vi "Remove Routing and Faulting Custom Device.vi"(8 "error in":errorcluster, 11 "routing and faulting custom device":T1 format="%.0x") -> (0 "error out":errorcluster)   [LabVIEW 2020, in "Routing and Faulting Scripting.lvlib"]
doc: "Removes the Routing and Faulting custom device from its parent. This removes all routing channels and endpoint aliases."
uses:
  Routing and Faulting Scripting.lvlib
  <vilib>/NI VeriStand/Custom Device API/Custom Device Item Ref.ctl
  NationalInstruments.VeriStand.SystemDefinitionAPI
  <vilib>/NI VeriStand/Custom Device API/Custom Device API.lvlib
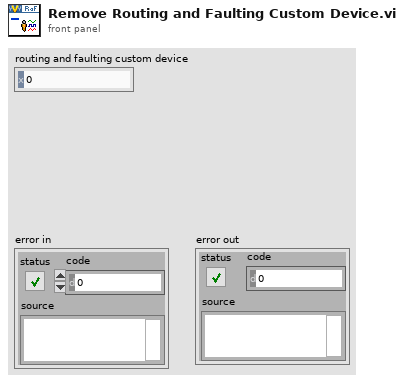
[diagram p1: front panel]
types:
  T1 = typedef "Custom Device API.lvlib/Custom Device Item Ref.ctl" = u64
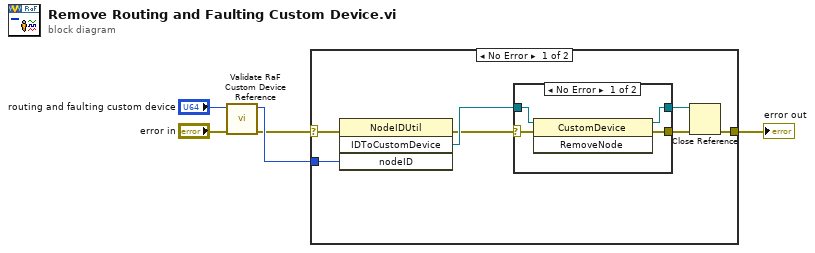
[diagram p0: block diagram]
diagram:
  n1 = call "Validate RaF Custom Device Reference.vi"("error in"="error in", "routing and faulting in"="routing and faulting custom device") -> ("error out"=w1:errorcluster, "routing and faulting out"=w3:T1)  [unwired: 8 in]
  n2 = case shown="No Error" w1 {
    selector: w1 -> [w7 w19]
    tunnel: [w10 w19] -> w5
    tunnel: w3 -> [w8 _]
    frame No Error {
      n3 = invoke class="NodeIDUtil" method="IDToCustomDevice"(error in=w7, "nodeID"=w8) -> (error out=w6:errorcluster, "IDToCustomDevice"=w9:refnum<k24>)  [unwired: 2 in, 2 out]
      n4 = case shown="No Error" w6 {
        selector: w6 -> [w15 w18]
        tunnel: w9 -> [w16 w17]
        tunnel: [w14 w17] -> w12
        tunnel: [w13 w18] -> w11
        frame No Error {
          n5 = invoke class="CustomDevice" method="RemoveNode"(reference=w16, error in=w15) -> (reference out=w14:refnum<k24>, error out=w13:errorcluster)  [unwired: 1 in, 1 out]
        }
        frame Error {
        }
      }
      n6 = Close Reference(reference=w12, error in (no error)=w11) -> (error out=w10:errorcluster)
    }
    frame Error {
    }
  }
  "error out" <- w5
